vi "Save Plugin Setup String.vi"(2 "Plug In Pathname":path, 3 "Setup String to Save":string, 4 "PlugIn Label":string) -> (0 "Meas Setup File":bool, 1 "Raw Data File Written to":path[](array[path]))   [LabVIEW 2022 SP3]
uses:
  File/Setup_Filetype.ctl
  Globals/Meas_global.vi
  Data_plotting_vis/Results_plotter_Global.vi
panel:
  out "name":string
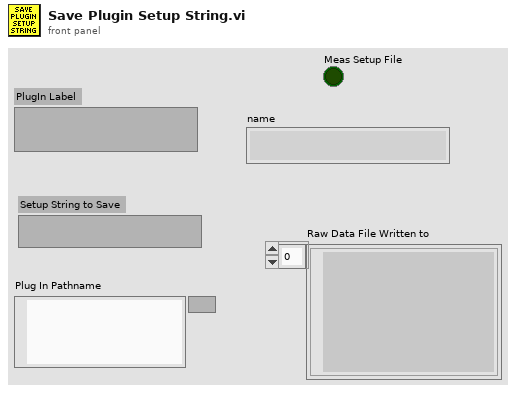
[diagram p1: front panel]
types:
  T1 = typedef "Setup_Filetype.ctl" = enum16{"Measurement Setups", "Calibration Setups", "General", "Results File Plotter Setups", "Speed Calib Tweaks"}
  T2 = enum16{"Zero or one", "One", "Zero or more", "One or more"}
  T3 = typedef "Post_Process.ctl" = enum16{"Take New Data", "Post Process Raw Data File"}
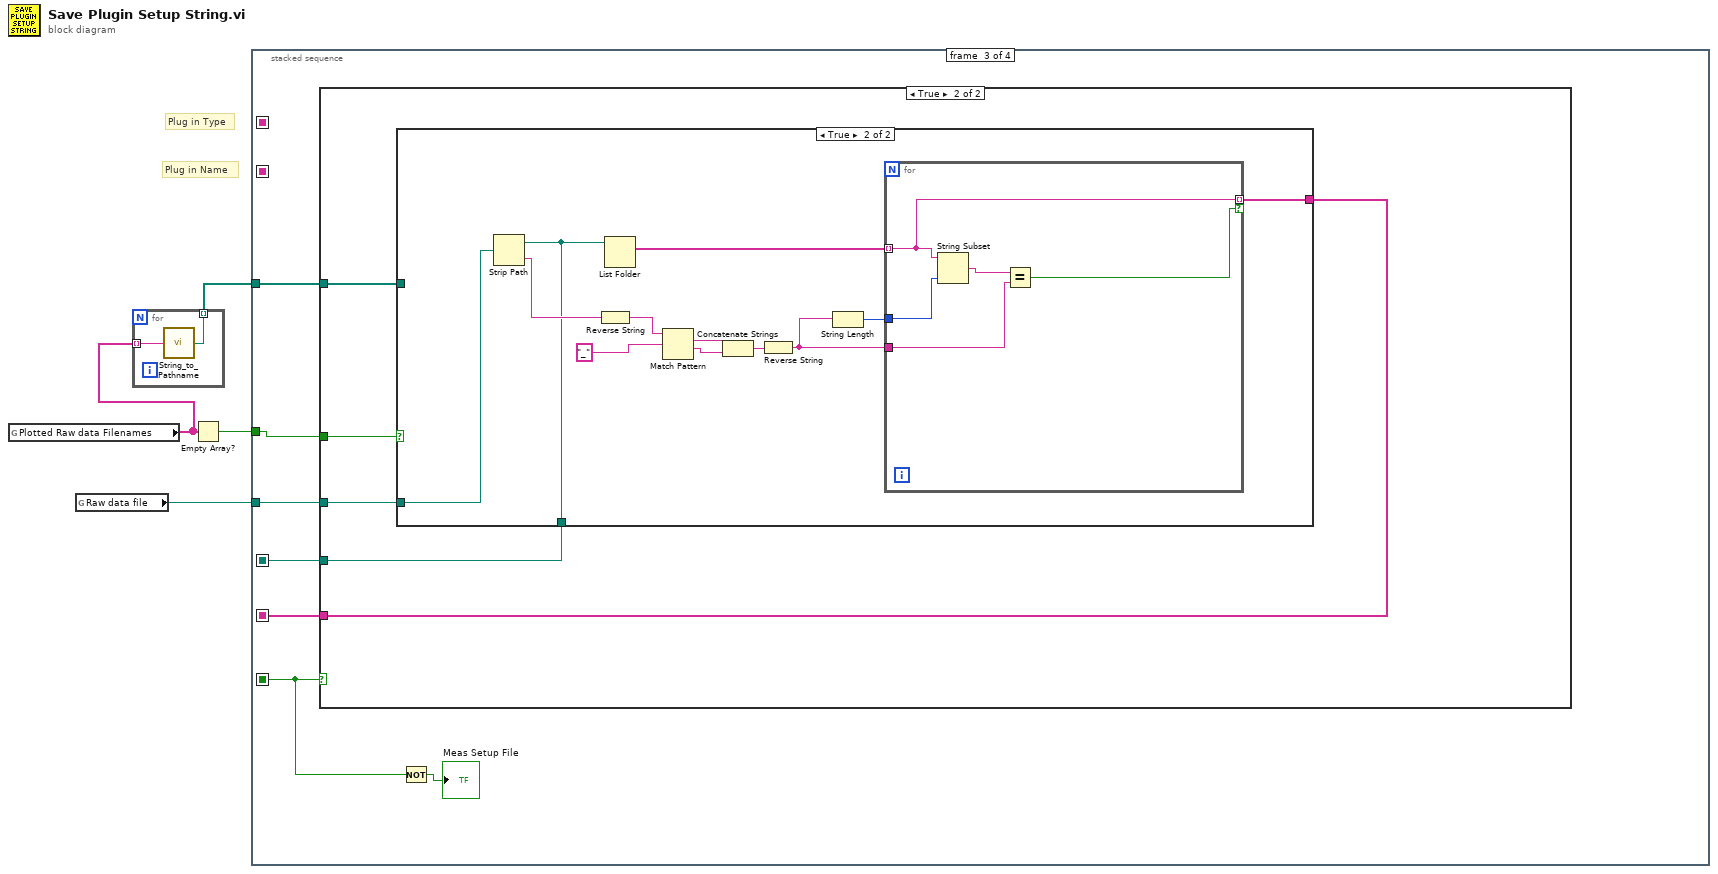
[diagram p0: block diagram]
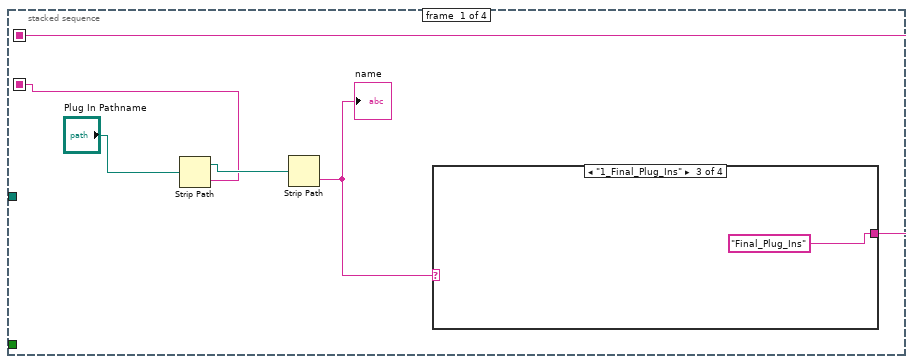
[diagram p2: hidden frame]
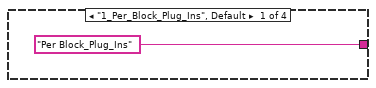
[diagram p3: hidden frame]
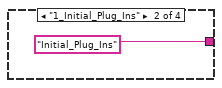
[diagram p4: hidden frame]
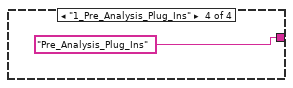
[diagram p5: hidden frame]
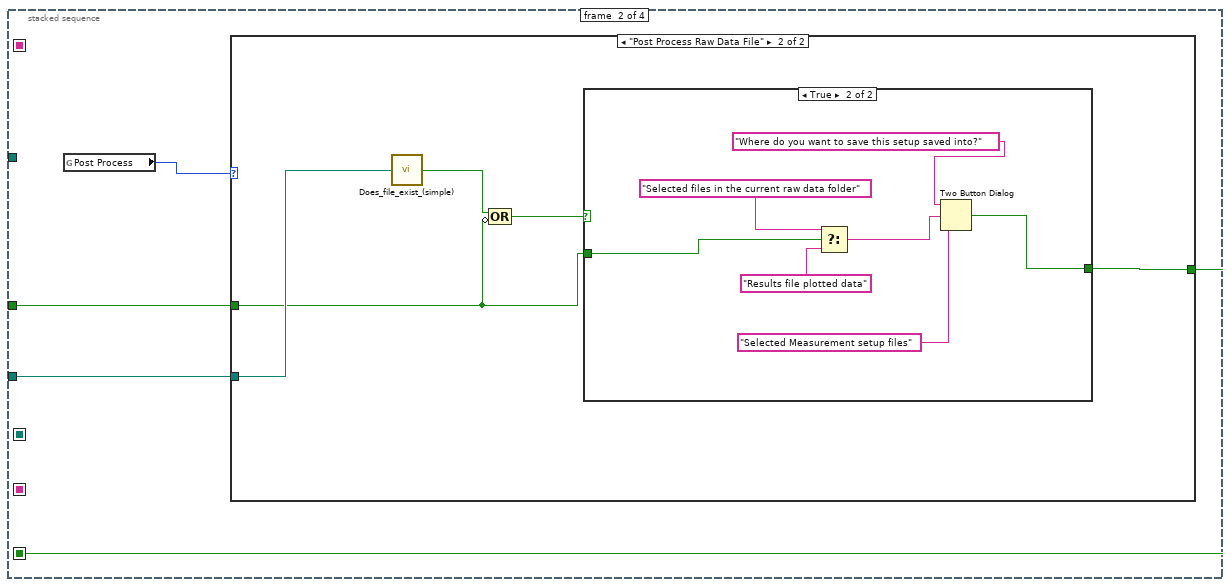
[diagram p6: hidden frame]
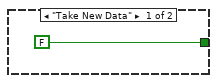
[diagram p7: hidden frame]
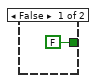
[diagram p8: hidden frame]
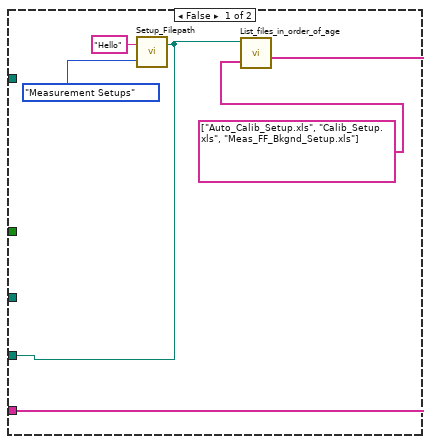
[diagram p9: hidden frame]
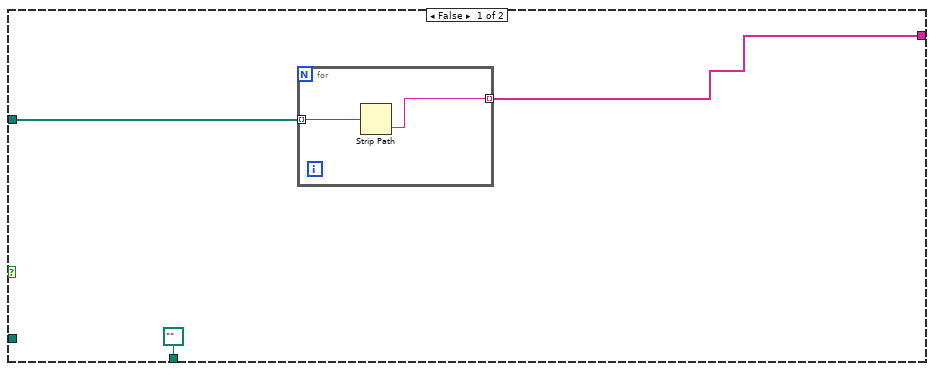
[diagram p10: hidden frame]
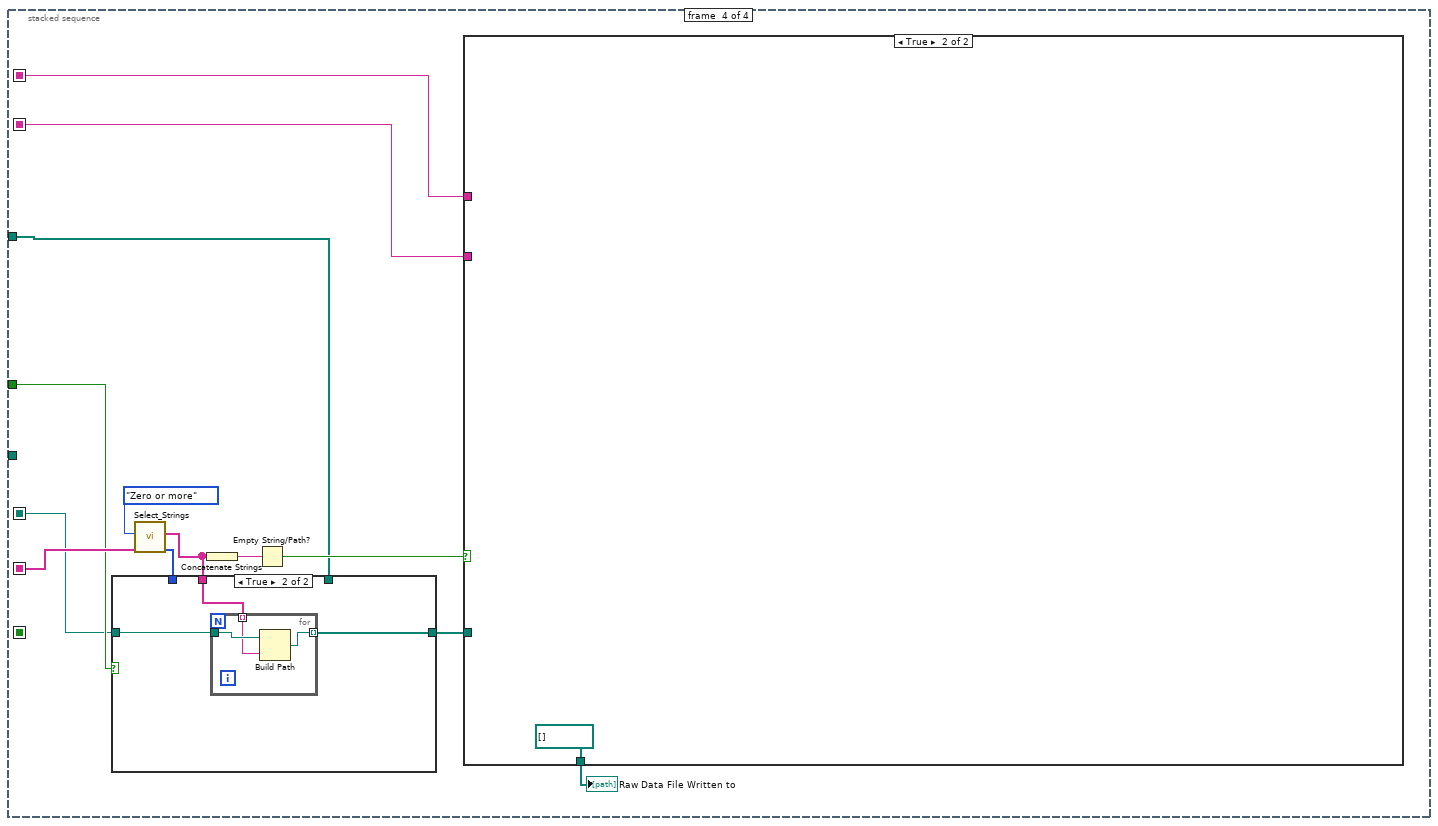
[diagram p11: hidden frame]
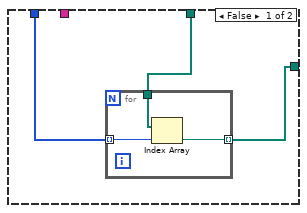
[diagram p12: hidden frame]
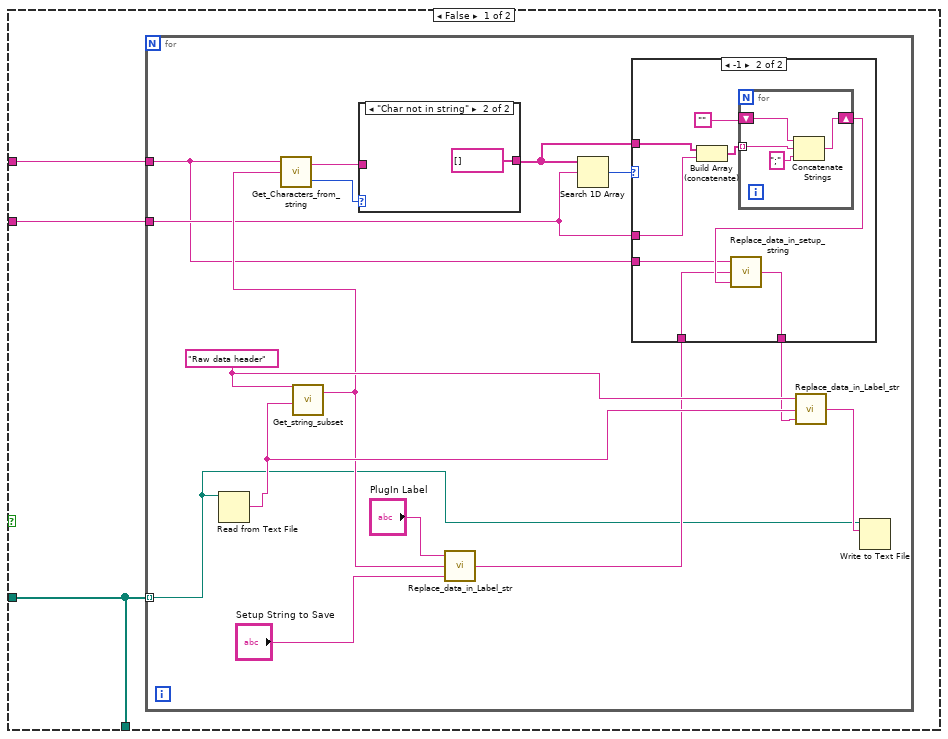
[diagram p13: hidden frame]
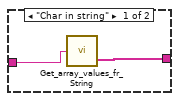
[diagram p15: hidden frame]
diagram:
  # "Plug in Name"
  # "Plug in Type"
  n1 = global read "Results_plotter_Global.vi" "Plotted Raw data Filenames"() -> (w2:string[])
  n2 = global read "Meas_global.vi" "Raw data file"() -> (w4:path)
  n3 = for {
    tunnel: w2 -> [w6] mode=indexing
    tunnel: [w5] -> w1 mode=indexing
    n4 = call "String_to_Pathname.vi"("Input String"=w6) -> ("path"=w5:path)
  }
  n5 = Empty Array?(array=w2) -> (empty?=w3:bool)
  n6 = stacked-sequence {
    seq-local: [_ w18 _ _] -> [_ _ w35 _]
    seq-local: [_ _ w40 _] -> [_ _ _ w82]
    seq-local: [w8 _ _ _] -> [_ _ _ w81]
    seq-local: [w7 _ _ _] -> [_ _ _ w80]
    seq-local: [_ _ w36 _] -> [_ _ _ w75]
    tunnel: w4 -> [_ w17 w37 _]
    tunnel: w3 -> [_ w16 w39 w79]
    tunnel: w1 -> [_ _ w38 w76]
    frame #0 {
      n7 = Strip Path(path="Plug In Pathname") -> (stripped path=w10:path, name=w7:string)
      n8 = Strip Path(path=w10) -> (name=w9:string)  [unwired: 1 out]
      "name" <- w9
      n9 = case shown="\"1_Final_Plug_Ins\"" w9 {
        tunnel: ["Per Block_Plug_Ins" "Initial_Plug_Ins" "Final_Plug_Ins" "Pre_Analysis_Plug_Ins"] -> w8
        frame "1_Per_Block_Plug_Ins", Default {
        }
        frame "1_Initial_Plug_Ins" {
        }
        frame "1_Final_Plug_Ins" {
        }
        frame "1_Pre_Analysis_Plug_Ins" {
        }
      }
    }
    frame #1 {
      n10 = global read "Meas_global.vi" "Post Process"() -> (w19:T3)
      n11 = case shown="\"Post Process Raw Data File\"" w19 {
        tunnel: [FALSE ("true") w25] -> w18
        tunnel: w17 -> [_ w24]
        tunnel: w16 -> [_ w21]
        frame "Take New Data" {
        }
        frame "Post Process Raw Data File" {
          n12 = call "Does_file_exist_(simple).vi"("Pathname"=w24) -> ("exists?"=w23:bool)
          n13 = Compound Arithmetic op=OR(w23, invert w21) -> (w22:bool)
          n14 = case shown="True" w22 {
            tunnel: [FALSE ("true") w33] -> w25
            tunnel: w21 -> [_ w30]
            frame False {
            }
            frame True {
              n15 = Select(t="Selected files in the current raw data folder" ("T button name (\"OK\")"), s=w30, f="Results file plotted data" ("T button name (\"OK\")")) -> (s? t:f=w27:string)
              n16 = Two Button Dialog(message="Where do you want to save this setup saved into?", 1:"Selected Measurement setup files" ("T button name (\"OK\")"), 2:w27) -> (T button?=w33:bool)
            }
          }
        }
      }
    }
    frame #2 {
      n17 = case shown="True" w35 {
        tunnel: [w42 w50] -> w40
        tunnel: w39 -> [_ w49]
        tunnel: w38 -> [_ w48]
        tunnel: w37 -> [_ w47]
        tunnel: [w41 w46] -> w36
        frame False {
          n18 = call "Setup_Filepath.vi"("Setup File Type"=Setup_Filetype."Measurement Setups", "Filename in"="Hello") -> ("Directory"=w41:path)  [unwired: 1 out]
          n19 = call "List_files_in_order_of_age.vi"("Files to Hide"=string[] ["Auto_Calib_Setup.xls", "Calib_Setup.xls", "Meas_FF_Bkgnd_Setup.xls"] ("file names"), "Folder"=w41) -> ("file names"=w42:string[])  [unwired: 9 in]
        }
        frame True {
          n20 = case shown="True" w49 {
            tunnel: [w52 w61] -> w50
            tunnel: w48 -> [w53 _]
            tunnel: w47 -> [_ w57]
            tunnel: [path "" ("stripped path") w56] -> w46
            frame False {
              n21 = for {
                tunnel: w53 -> [w55] mode=indexing
                tunnel: [w54] -> w52 mode=indexing
                n22 = Strip Path(path=w55) -> (name=w54:string)  [unwired: 1 out]
              }
            }
            frame True {
              n23 = Strip Path(path=w57) -> (stripped path=w56:path, name=w67:string)
              n24 = Reverse String(1:w67) -> (0:w66:string)
              n25 = List Folder(path=w56) -> (filenames=w63:string[])  [unwired: 3 in, 3 out]
              n26 = Match Pattern(string=w66, regular expression="_") -> (match substring=w60:string, after substring=w59:string)  [unwired: 1 in, 2 out]
              n27 = Concatenate Strings(w60, w59) -> (w58:string)
              n28 = Reverse String(1:w58) -> (0:w62:string)
              n29 = String Length(string=w62) -> (length=w64:i32)
              n30 = for {
                tunnel: w64 -> [w72]
                tunnel: w63 -> [w69] mode=indexing
                tunnel: w62 -> [w70]
                tunnel: [w69] -> w61 mode=indexing if=w68
                n31 = String Subset(string=w69, length (rest)=w72) -> (substring=w71:string)  [unwired: 1 in]
                n32 = Equal?(x=w71, y=w70) -> (x = y?=w68:bool)
              }
            }
          }
        }
      }
      n33 = Not(x=w35) -> (.not. x?=→"Meas Setup File":bool)
    }
    frame #3 {
      n34 = call "Select_Strings.vi"("Available Ch names"=w82, "Selector mode"=T2."Zero or more") -> ("Ch Indicies Chosen"=w74:i32[], "Selected Channel Names"=w78:string[])  [unwired: 4 in, 1 out]
      n35 = case shown="True" w79 {
        tunnel: w78 -> [_ w94]
        tunnel: [w86 w93] -> w77
        tunnel: w76 -> [w88 _]
        tunnel: w75 -> [_ w92]
        tunnel: w74 -> [w87 _]
        frame False {
          n36 = for {
            tunnel: w88 -> [w91]
            tunnel: w87 -> [w90] mode=indexing
            tunnel: [w89] -> w86 mode=indexing
            n37 = Index Array(array=w91, index=w90) -> (element=w89:path)
          }
        }
        frame True {
          n38 = for {
            tunnel: w92 -> [w97]
            tunnel: w94 -> [w96] mode=indexing
            tunnel: [w95] -> w93 mode=indexing
            n39 = Build Path(base path=w97, name or relative path=w96) -> (appended path=w95:path)
          }
        }
      }
      n40 = Concatenate Strings(w78) -> (w83:string)
      n41 = Empty String/Path?(string/path=w83) -> (empty?=w84:bool)
      n42 = case shown="True" w84 {
        tunnel: w77 -> [w98 _]
        tunnel: w81 -> [w100 _]
        tunnel: w80 -> [w99 _]
        tunnel: [w98 path[] []] -> w73
        frame False {
          n43 = for {
            tunnel: w98 -> [w101] mode=indexing
            tunnel: w100 -> [w102]
            tunnel: w99 -> [w105]
            w113 = "Raw data header"
            n44 = Read from Text File(file (use dialog)=w101) -> (text=w115:string)  [unwired: 3 in, 3 out]
            n45 = call "Get_string_subset.vi"("String to split"=w115, "File Label"=w113) -> ("Output string"=w110:string)  [unwired: 2 in, 1 out]
            n46 = call "Get_Characters_from_string.vi"("Input string"=w110, "Variable name"=w102) -> ("Status"=w109:enum16{"Char in string", "Char not in string"}, "Value"=w108:string)  [unwired: 1 in]
            n47 = case shown="\"Char not in string\"" w109 {
              tunnel: [w130 string[] [] ("String array")] -> w106
              tunnel: w108 -> [w129 _]
              frame "Char in string" {
                n48 = call "Get_array_values_fr_String.vi"("String Value"=w129) -> ("String array"=w130:string[])  [unwired: 1 out]
              }
              frame "Char not in string" {
              }
            }
            n49 = call "Replace_data_in_Label_str.vi"("New data string"="Setup String to Save", "Input string"=w110, "Variable name"="PlugIn Label") -> ("Appended string"=w104:string)
            n50 = Search 1D Array(1D array=w106, element=w105) -> (index of element=w107:i32)  [unwired: 1 out]
            n51 = case shown="-1" w107 {
              tunnel: w106 -> [_ w124]
              tunnel: w105 -> [_ w123]
              tunnel: w104 -> [w116 w119]
              tunnel: [w116 w117] -> w103
              tunnel: w102 -> [_ w118]
              frame 0, Default {
              }
              frame -1 {
                n52 = Build Array (concatenate)(w124, w123) -> (w122:string[])
                n53 = for {
                  shift-right: [w126] -> w120
                  shift-left: "" -> [w127]
                  tunnel: w122 -> [w125] mode=indexing
                  n54 = Concatenate Strings(w127, w125, ";" ("string")) -> (w126:string)
                }
                n55 = call "Replace_data_in_setup_string.vi"("New data string"=w120, "Input string"=w119, "Variable name"=w118) -> ("Appended string"=w117:string)
              }
            }
            n56 = call "Replace_data_in_Label_str.vi"("New data string"=w103, "Input string"=w115, "Variable name"=w113) -> ("Appended string"=w114:string)
            n57 = Write to Text File(file (use dialog)=w101, text=w114) -> ()  [unwired: 2 in, 3 out]
          }
        }
        frame True {
        }
      }
      "Raw Data File Written to" <- w73
    }
  }
